vi "Z Settings.vi"(8 "error in (no error)":errorcluster, 11 "Dispense in":refnum<class "Dispense.lvclass">) -> (0 "error out":errorcluster, 3 "Dispense out":refnum<class "Dispense.lvclass">)   [LabVIEW 2021, in "Dispense.lvclass"]
uses:
  Dispense.lvclass
  Dispense.lvclass/Dispense.ctl
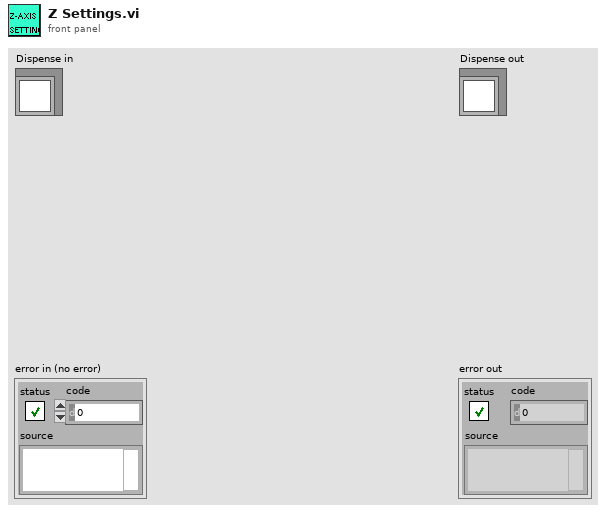
[diagram p1: front panel]
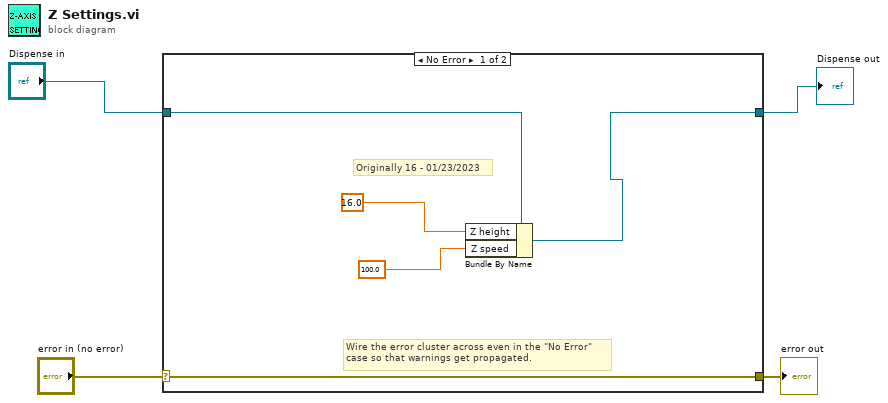
[diagram p0: block diagram]
diagram:
  n1 = case shown="No Error" "error in (no error)" {
    selector: "error in (no error)" -> [w9 w11]
    tunnel: [w9 w11] -> w3
    tunnel: [w5 w10] -> w1
    tunnel: "Dispense in" -> [w8 w10]
    frame No Error {
      # "Originally 16 - 01/23/2023"
      # "Wire the error cluster across even in the \"No Error\"\ncase so that warnings get propagated."
      n2 = Bundle By Name(cluster=w8, "Z height"=16.0, "Z speed"=100.0) -> (w5:refnum<class "Dispense.lvclass">)
    }
    frame Error {
    }
  }
  "error out" <- w3
  "Dispense out" <- w1
